vi "Acknowledge Faults.vi"(0 "reference in":refnum<class "Simulated-PowerModule.lvclass">, 11 "Error In":errorcluster) -> (4 "reference out":refnum<class "Simulated-PowerModule.lvclass">, 15 "Error Out":errorcluster)   [LabVIEW 2023, in "Simulated-PowerModule.lvlib" / "Simulated-PowerModule.lvclass"]
uses:
  Simulated-PowerModule.lvclass
  Simulated-PowerModule.lvclass/Simulated-PowerModule.ctl
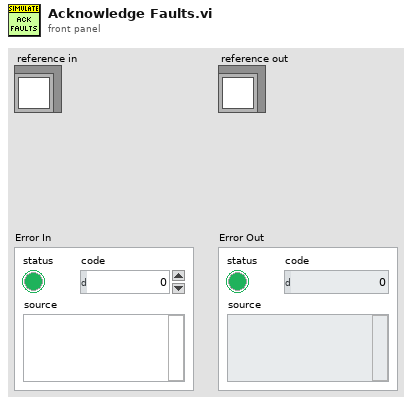
[diagram p1: front panel]
types:
  T1 = typedef "Simulated-PowerModule.lvlib/Simulated-PowerModule.lvclass/ObjectAttributes.ctl" = cluster{"JSON Config Path":path, "Configuration":T2, "connected":bool, "reserved":bool, "setpoint":cluster{"voltage":sgl, "current":sgl, "resistance":sgl}, "last timestamp":i64, "mode":T4, "range":T3, "measurement array":T5[]}
  T2 = typedef "Simulated-PowerModule.lvlib/Simulated-PowerModule.lvclass/Configuration.ctl" = cluster{"range":T3}
  T3 = typedef "PowerModuleInterface.lvlibp/PowerModuleInterface.lvclass/Range.ctl" = cluster{"Current Max (A)":dbl, "Current Min (A)":dbl, "Voltage Max (V)":dbl, "Voltage Min (V)":dbl}
  T4 = typedef "Simulated-PowerModule.lvlib/Simulated-PowerModule.lvclass/Mode.ctl" = u16
  T5 = typedef "PowerModuleInterface.lvlibp/PowerModuleInterface.lvclass/Measurements.ctl" = cluster{"measured voltage (V)":dbl, "measured current (A)":dbl, "setpoint voltage (V)":dbl, "setpoint current (A)":dbl, "timestamp":dbl}
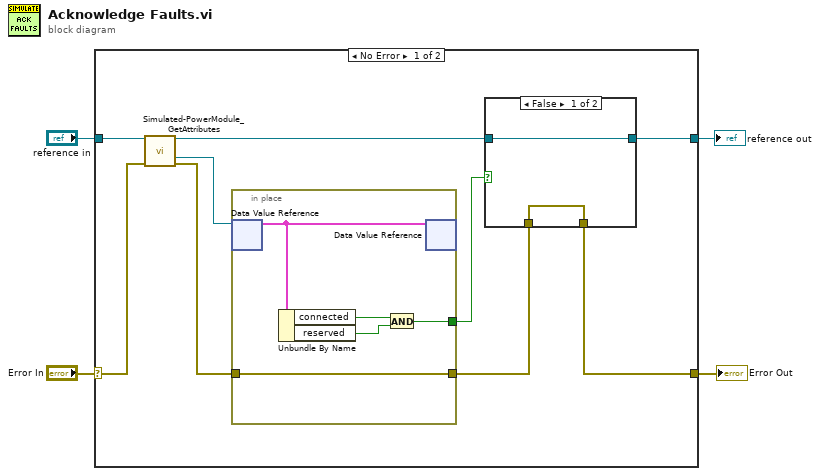
[diagram p0: block diagram]
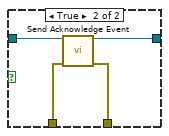
[diagram p2: hidden frame]
diagram:
  n1 = case shown="No Error" "Error In" {
    selector: "Error In" -> [w12 w25]
    tunnel: "reference in" -> [w13 w26]
    tunnel: [w7 w26] -> w4
    tunnel: [w6 w25] -> w2
    frame No Error {
      n2 = call "Simulated-PowerModule_GetAttributes.vi"("reference in"=w13, "Error In"=w12) -> ("reference out"=w8:refnum<class "Simulated-PowerModule.lvclass">, "DataRef"=w11:refnum<data-value>, "Error Out"=w10:errorcluster)  [unwired: 10 in, 1 out]
      n3 = in-place {
        in-place-border: w10 -> [w24]
        in-place-border: [w24] -> w9
        in-place-border: [w20] -> w5
        n4 = in-place-dvr #1(w11) -> (w21:T1)  [unwired: 1 out]
        n5 = Unbundle By Name(w21) -> ("connected"=w23:bool, "reserved"=w22:bool)
        n6 = And(x=w23, y=w22) -> (x .and. y?=w20:bool)
        n7 = in-place-dvr #1(w21) -> ()  [unwired: 2 out]
      }
      n8 = case shown="False" w5 {
        tunnel: w9 -> [w14 w19]
        tunnel: w8 -> [w15 w18]
        tunnel: [w15 w17] -> w7
        tunnel: [w14 w16] -> w6
        frame False {
        }
        frame True {
          n9 = call "Send Acknowledge Event.vi"("reference in"=w18, "Error In"=w19) -> ("reference out"=w17:refnum<class "Simulated-PowerModule.lvclass">, "Error Out"=w16:errorcluster)  [unwired: 12 in]
        }
      }
    }
    frame Error {
    }
  }
  "Error Out" <- w2
  "reference out" <- w4
